vi "Recieve Acknowledge Initialized.vi"(8 "error in (no error)":errorcluster, 9 "Requestor":string, 10 "Requestee":string, 11 "Meter Measurement in":refnum<class "Meter Measurement.lvclass">) -> (0 "error out":errorcluster, 3 "Meter Measurement out":refnum<class "Meter Measurement.lvclass">)   [LabVIEW 2015, in "Meter Measurement.lvclass"]
uses:
  Meter Measurement.lvclass
  Mag Lab Root/Mag Lab Root.lvclass/Mag Lab Root.ctl
  Meter Measurement.lvclass/Meter Measurement.ctl
  <vilib>/ActorFramework/Actor/Actor.lvclass/Actor.ctl
  Mag Lab Root Messages/Recieve Acknowledge Initialized Msg/Recieve Acknowledge Initialized Msg.lvclass/Recieve Acknowledge Initialized Msg.ctl
  <vilib>/ActorFramework/Message Enqueuer/Message Enqueuer.lvclass/Message Enqueuer.ctl
  <vilib>/ActorFramework/Message Enqueuer/Enqueue.vi
  <vilib>/ActorFramework/Message Priority Queue/Priority Enqueue.vi
  Mag Lab Root Messages/Recieve Acknowledge Initialized Msg/Recieve Acknowledge Initialized Msg.lvclass
  Mag Lab Root/Mag Lab Root.lvclass
  <vilib>/ActorFramework/Actor/Actor.lvclass
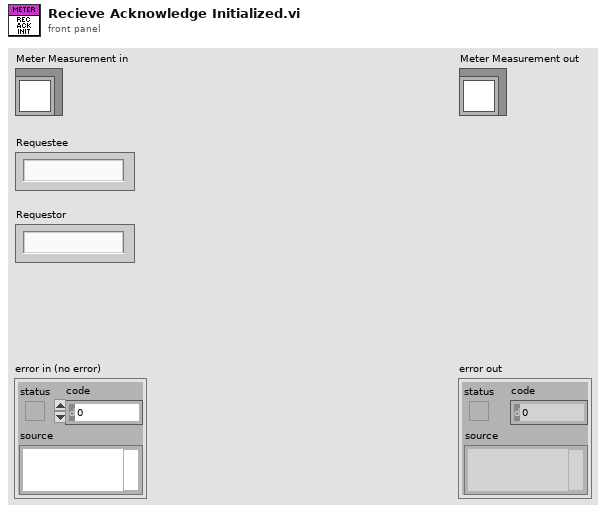
[diagram p1: front panel]
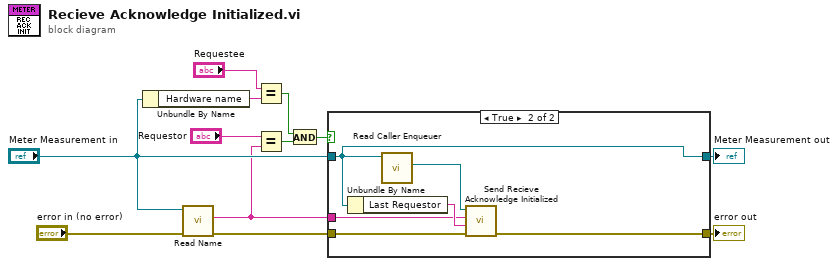
[diagram p0: block diagram]
diagram:
  n1 = Unbundle By Name("Meter Measurement in") -> ("Hardware name"=w11:string)
  n2 = call "Read Name.vi"("error in (no error)"="error in (no error)", "Mag Lab Root in"="Meter Measurement in") -> ("error out"=w6:errorcluster, "Name"=w2:string)  [unwired: 7 in, 1 out]
  n3 = Equal?(x="Requestee", y=w11) -> (x = y?=w10:bool)
  n4 = Equal?(x="Requestor", y=w2) -> (x = y?=w9:bool)
  n5 = And(x=w10, y=w9) -> (x .and. y?=w8:bool)
  n6 = case shown="True" w8 {
    tunnel: "Meter Measurement in" -> [w13 w15]
    tunnel: w2 -> [_ w17]
    tunnel: w6 -> [w14 w20]
    tunnel: [w14 w16] -> w4
    tunnel: [w13 w15] -> w3
    frame False {
    }
    frame True {
      n7 = Unbundle By Name(w15) -> ("Last Requestor"=w18:string)
      n8 = call <vilib>:"Read Caller Enqueuer.vi"("Actor"=w15) -> ("Caller Enqueuer"=w19:refnum<class "Message Enqueuer.lvclass">)  [unwired: 10 in]
      n9 = call "Send Recieve Acknowledge Initialized.vi"("error in (no error)"=w20, "Requestor"=w18, "Requestee"=w17, "Message Enqueuer"=w19) -> ("error out"=w16:errorcluster)  [unwired: 6 in, 1 out]
    }
  }
  "error out" <- w4
  "Meter Measurement out" <- w3
